vi "Dig.vi"(6 "Variant in":variant, 7 "Shift Pressed?":bool, 8 "error in (no error)":errorcluster, 10 "QD Combo Box Ref":refnum<vi>, 11 "QD Launch VI Ref":refnum<vi>) -> (0 "error out":errorcluster, 4 "Variant out":variant)   [LabVIEW 2017, in "Quick Drop.lvlib"]
doc: "Digs a grave for the currently selected code. A grave is a Diagram Disable Structure with a bookmark for the structure label that includes \"RIP\", the time of death (YYYYMMDD), and the grave digger (programmer). The selected code is placed in the Disabled frame, which will have the \"Corpse\" subdiagram label and a duplicate of the Disabled frame is created for the Enabled frame, which will have the \"Spirit\" subdiagram label. The spirit of the original, legacy code can then be safely refactored.\n\nDefault Shortcut - [G]"
uses:
  Quick Drop.lvlib
  Toolkit/Toolkit.lvlib
panel:
  in  "Undo Name":string="Dig Grave"
  # "Do not change the connector pane of this VI.\n\nSee the block diagram for directions on how to use this template."
  # "Specify the name of the Undo transaction"
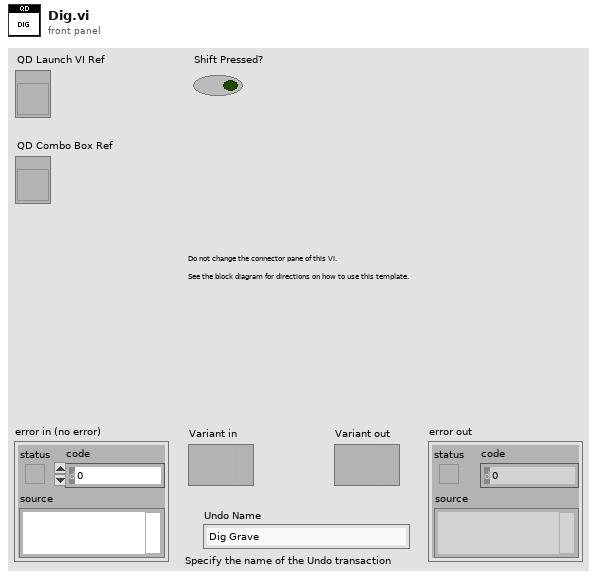
[diagram p1: front panel]
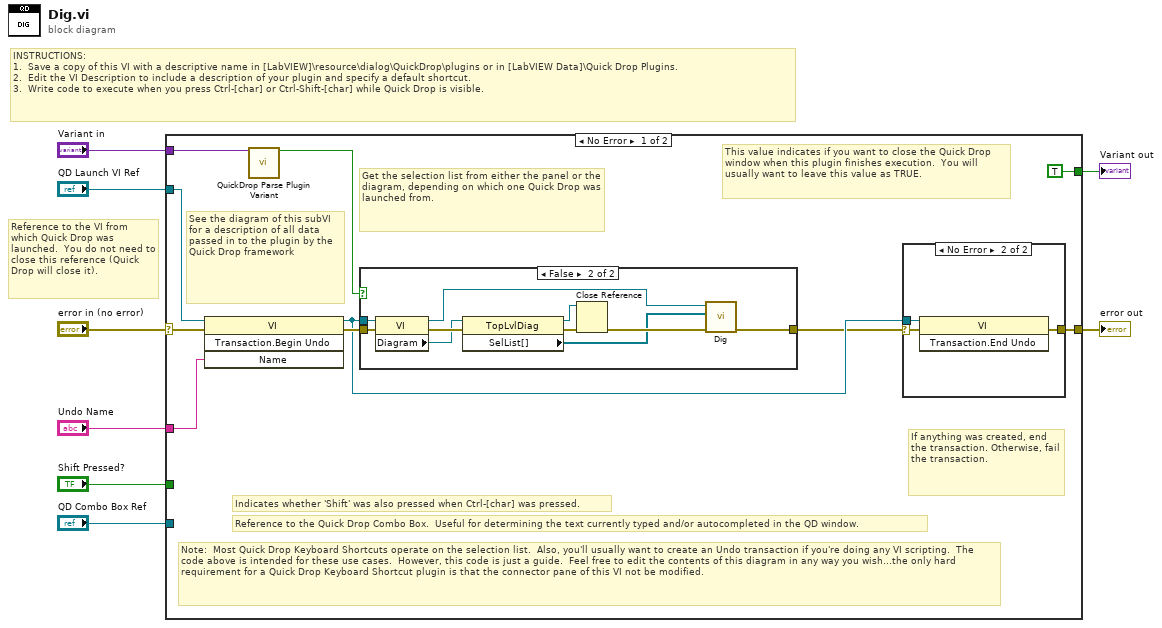
[diagram p0: block diagram]
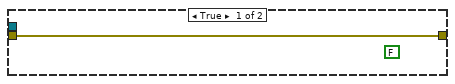
[diagram p2: hidden frame]
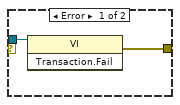
[diagram p3: hidden frame]
diagram:
  # "Reference to the VI from which Quick Drop was launched.  You do not need to close this reference (Quick Drop will close it)."
  # "INSTRUCTIONS:\n1.  Save a copy of this VI with a descriptive name in [LabVIEW]\\resource\\dialog\\QuickDrop\\plugins or in [LabVIEW Data]\\Quick Drop Plugins.\n2.  Edit the VI Description to include a description of your plugin and specify a default shortcut. \n3.  Write code to execute when you press Ctrl-[char] or Ctrl-Shift-[char] while Quick Drop is visible."
  n1 = case shown="No Error" "error in (no error)" {
    selector: "error in (no error)" -> [w17 w35]
    tunnel: [w11 w35] -> w7
    tunnel: "QD Launch VI Ref" -> [w16 _]
    tunnel: "Shift Pressed?" -> [_ _]
    tunnel: "QD Combo Box Ref" -> [_ _]
    tunnel: "Variant in" -> [w18 _]
    tunnel: "Undo Name" -> [w15 _]
    tunnel: [TRUE _] -> w1
    frame No Error {
      # "Note:  Most Quick Drop Keyboard Shortcuts operate on the selection list.  Also, you'll usually want to create an Undo transaction if you're doing any VI scripting.  The code above is intended for these use cases.  However, this code is just a guide.  Feel free to edit the contents of this diagram in any way you wish...the only hard requirement for a Quick Drop Keyboard Shortcut plugin is that the connector pane of this VI not be modified."
      # "Get the selection list from either the panel or the diagram, depending on which one Quick Drop was launched from."
      # "If anything was created, end the transaction. Otherwise, fail the transaction."
      # "This value indicates if you want to close the Quick Drop window when this plugin finishes execution.  You will usually want to leave this value as TRUE."
      # "See the diagram of this subVI for a description of all data passed in to the plugin by the Quick Drop framework"
      # "Reference to the Quick Drop Combo Box.  Useful for determining the text currently typed and/or autocompleted in the QD window."
      # "Indicates whether 'Shift' was also pressed when Ctrl-[char] was pressed."
      n2 = invoke class="VI" method="Transaction.Begin Undo"(reference=w16, error in=w17, "Name"=w15) -> (reference out=w10:refnum<vi>, error out=w12:errorcluster)  [unwired: 1 in, 2 out]
      n3 = call <vilib>:"QuickDrop Parse Plugin Variant.vi"("QDKS Variant in"=w18) -> ("QD Launch VI Panel?"=w13:bool)  [unwired: 12 in, 2 out]
      n4 = case shown="False" w13 {
        tunnel: w12 -> [w19 w29]
        tunnel: w10 -> [_ w22]
        tunnel: [w19 w21] -> w9
        frame True {
          (unwired) FALSE ("Change Made?")
        }
        frame False {
          n5 = property class="VI"(reference=w22, error in=w29) -> (reference out=w20:refnum<vi>, error out=w28:errorcluster, "Diagram"=w27:refnum<vi>)
          n6 = property class="TopLvlDiag"(reference=w27, error in=w28) -> (reference out=w25:refnum<vi>, error out=w26:errorcluster, "SelList[]"=w23:refnum<vi>[])
          n7 = Close Reference(reference=w25, error in (no error)=w26) -> (error out=w24:errorcluster)
          n8 = call "Dig.vi"("Error In"=w24, "Selection List[]"=w23, "VI In"=w20) -> ("Error Out"=w21:errorcluster)  [unwired: 7 in, 1 out]
        }
      }
      n9 = case shown="No Error" w9 {
        selector: w9 -> [_ w32]
        tunnel: [w31 w34] -> w11
        tunnel: w10 -> [w30 w33]
        frame Error {
          n10 = invoke class="VI" method="Transaction.Fail"(reference=w30) -> (error out=w31:errorcluster)  [unwired: 2 in, 2 out]
        }
        frame No Error {
          n11 = invoke class="VI" method="Transaction.End Undo"(reference=w33, error in=w32) -> (error out=w34:errorcluster)  [unwired: 1 in, 2 out]
        }
      }
    }
    frame Error {
    }
  }
  "error out" <- w7
  "Variant out" <- w1
